vi "Perform Action.vi"(8 "error in (no error)":errorcluster, 10 "Input":variant, 11 "Sample PID Light in":refnum<class "Sample PID Light.lvclass">) -> (0 "error out":errorcluster, 2 "Output":variant, 3 "Sample PID Light out":refnum<class "Sample PID Light.lvclass">)   [LabVIEW 2023, in "Sample PID Light.lvclass"]
uses:
  Sample PID Light.lvclass
  Sample PID Light.lvclass/Sample PID Light.ctl
  Task/Task Base/Task Base.lvclass
  Measure and Stimulus Subsystems/Measure and Stimulus Subsystems.lvclass
  <vilib>/addons/control/pid/NI_PID_pid.lvlib
  D:/git/HAL/HAL GOOP4/Task/Task Base/Task Base.lvclass
  D:/git/HAL/HAL GOOP4/Tests/Sample Tasks/Sample PID Light/Sample PID Light.lvclass
  <vilib>/addons/control/pid/pid.llb/PID (DBL).vi
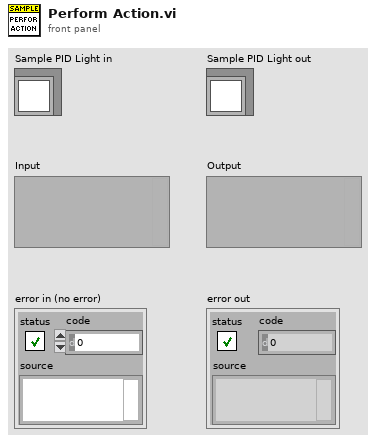
[diagram p1: front panel]
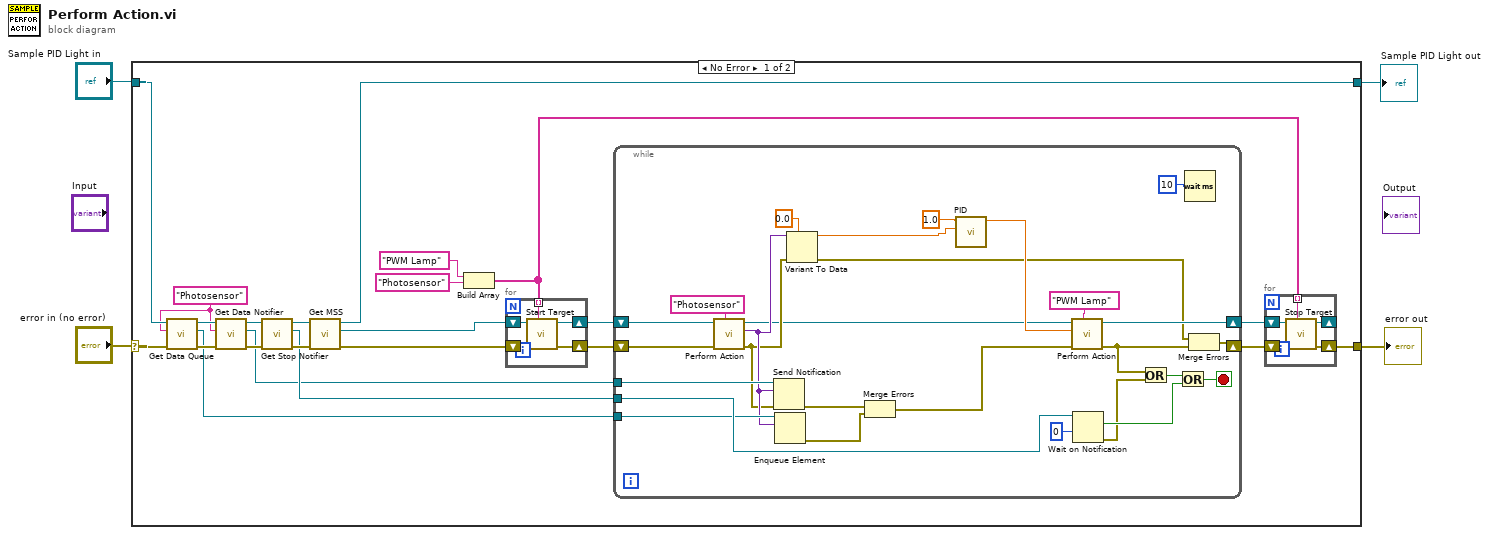
[diagram p0: block diagram]
diagram:
  n1 = case shown="No Error" "error in (no error)" {
    selector: "error in (no error)" -> [w24 w66]
    tunnel: [w20 w66] -> w2
    tunnel: [w11 w65] -> w1
    tunnel: "Sample PID Light in" -> [w13 w65]
    frame No Error {
      w5 = "Photosensor" ("Name")
      n2 = call "Get Data Queue.vi"("error in (no error)"=w24, "Name"=w5, "Task Base in"=w13) -> ("error out"=w14:errorcluster, "Data Queue"=w12:refnum<queue>, "Task Base out"=w8:refnum<class "Sample PID Light.lvclass">)  [unwired: 6 in]
      n3 = call "Get Data Notifier.vi"("error in (no error)"=w14, "Name"=w5, "Task Base in"=w8) -> ("error out"=w9:errorcluster, "Data Notifier"=w6:refnum<notifier>, "Task Base out"=w7:refnum<class "Sample PID Light.lvclass">)  [unwired: 6 in]
      n4 = call "Get Stop Notifier.vi"("error in (no error)"=w9, "Task Base in"=w7) -> ("error out"=w19:errorcluster, "Stop PE"=w10:refnum<notifier>, "Task Base out"=w18:refnum<class "Sample PID Light.lvclass">)  [unwired: 7 in]
      n5 = call "Get MSS.vi"("error in (no error)"=w19, "Task Base in"=w18) -> ("error out"=w23:errorcluster, "MSS"=w22:refnum<class "Measure and Stimulus Subsystems.lvclass">, "Task Base out"=w11:refnum<class "Sample PID Light.lvclass">)  [unwired: 7 in]
      n6 = Build Array("PWM Lamp" ("Target Ident"), "Photosensor" ("Target Identifier")) -> (w15:string[])
      n7 = for {
        shift-right: [w32] -> w27
        shift-left: w23 -> [w30]
        shift-right: [w31] -> w26
        shift-left: w22 -> [w29]
        tunnel: w15 -> [w28] mode=indexing
        n8 = call "Start Target.vi"("Target Ident"=w28, "Error In"=w30, "reference in"=w29) -> ("Error Out"=w32:errorcluster, "reference out"=w31:refnum<class "Measure and Stimulus Subsystems.lvclass">)  [unwired: 7 in]
      }
      n9 = while {
        shift-right: [w50] -> w25
        shift-left: w27 -> [w55]
        shift-right: [w57] -> w21
        shift-left: w26 -> [w54]
        tunnel: w10 -> [w44]
        tunnel: w6 -> [w45]
        tunnel: w12 -> [w40]
        stop <- w48 stop-if-true
        n10 = call "Perform Action.vi"("Target Ident"="Photosensor" ("Target Identifier"), "Error In"=w55, "reference in"=w54) -> ("Error Out"=w34:errorcluster, "Output"=w35:variant, "reference out"=w33:refnum<class "Measure and Stimulus Subsystems.lvclass">)  [unwired: 6 in]
        n11 = Send Notification(notification=w35, notifier=w45, error in (no error)=w34) -> (error out=w37:errorcluster)  [unwired: 1 out]
        n12 = Enqueue Element(queue=w40, element=w35) -> (error out=w39:errorcluster)  [unwired: 2 in, 2 out]
        n13 = Variant To Data(error in=w34, type=0.0, Variant=w35) -> (data=w52:dbl, error out=w49:errorcluster)
        n14 = Merge Errors(w37, w39) -> (w38:errorcluster)
        n15 = call-poly <vilib>:"PID.vi"("process variable"=w52, "setpoint"=1.0) -> ("output"=w51:dbl)  [unwired: 8 in, 1 out]
        n16 = call "Perform Action.vi"("Target Ident"="PWM Lamp", "Error In"=w38, "Input"=w51, "reference in"=w33) -> ("Error Out"=w41:errorcluster, "reference out"=w57:refnum<class "Measure and Stimulus Subsystems.lvclass">)  [unwired: 5 in, 1 out]
        n17 = Wait on Notification(notifier=w44, timeout in ms (-1)=0) -> (notification=w46:bool, error out=w43:errorcluster)  [unwired: 2 in, 2 out]
        n18 = Or(x=w41, y=w43) -> (x .or. y?=w42:bool)
        n19 = Or(x=w42, y=w46) -> (x .or. y?=w48:bool)
        n20 = Wait (ms)(milliseconds to wait=u32 10) -> ()  [unwired: 1 out]
        n21 = Merge Errors(w49, w41) -> (w50:errorcluster)
      }
      n22 = for {
        shift-right: [w62] -> w20
        shift-left: w25 -> [w64]
        tunnel: w15 -> [w61] mode=indexing
        shift-right: [w60] -> _
        shift-left: w21 -> [w63]
        n23 = call "Stop Target.vi"("Target Ident"=w61, "Error In"=w64, "reference in"=w63) -> ("Error Out"=w62:errorcluster, "reference out"=w60:refnum<class "Measure and Stimulus Subsystems.lvclass">)  [unwired: 7 in]
      }
    }
    frame Error {
    }
  }
  "error out" <- w2
  "Sample PID Light out" <- w1
